vi "Auto Execute Commands.vi"(11 "Auto Commands":T1=[{"Drive Duration"=0.0, "Left Speed"=0.0, "Right Speed"=0.0, "Set Point"=1.0, "Set Point Duration"=2.0, "Command"=enum."Shooter", "Wait ms"=0.0}]) -> ()   [LabVIEW 2019]
uses:
  Controls/Auto Controls.ctl
  <vilib>/Rock Robotics/WPI/Solenoid/WPI_SolenoidValue.ctl
  <vilib>/Rock Robotics/WPI/Solenoid/WPI_SolenoidSetEnum.vi
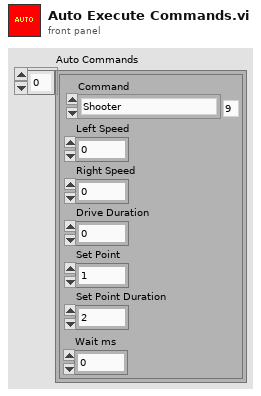
[diagram p1: front panel]
types:
  T1 = typedef "Auto Controls.ctl" = cluster{"Drive Duration":dbl, "Left Speed":dbl, "Right Speed":dbl, "Set Point":dbl, "Set Point Duration":dbl, "Command":enum16{"", "Drive Forwards", "Drive Backwards", "Stop", "Turn Left", "Turn Right", "Drop Intake", "Lift Intake", "Intake", "Shooter", "Transfer", "Wait"}, "Wait ms":dbl}[]
  T2 = typedef "WPI_SolenoidValue.ctl" = enum16{"Off", "On", "Forward", "Reverse"}
  T3 = enum16{"", "Drive Forwards", "Drive Backwards", "Stop", "Turn Left", "Turn Right", "Drop Intake", "Lift Intake", "Intake", "Shooter", "Transfer", "Wait"}
  T4 = typedef "WPI_SolenoidDevRef.ctl" = cluster{"DevStatus":errorcluster, "Pneumatics Control Module":u8, "Forward Solenoid Channel":T5, "Reverse Solenoid Channel":T5}
  T5 = typedef "WPI_SolenoidChannel.ctl" = enum8{"Solenoid 0", "Solenoid 1", "Solenoid 2", "Solenoid 3", "Solenoid 4", "Solenoid 5", "Solenoid 6", "Solenoid 7", "Invalid"}
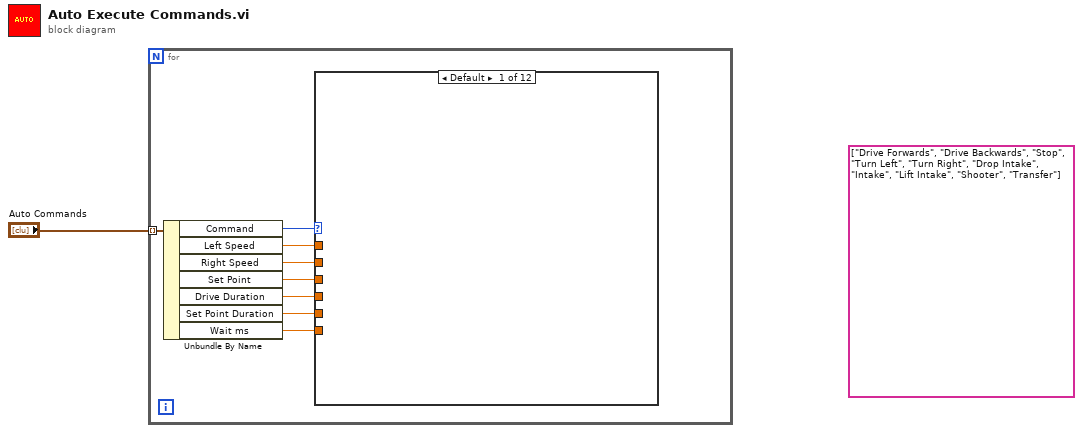
[diagram p0: block diagram]
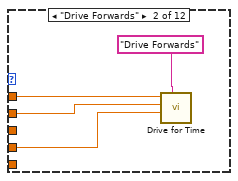
[diagram p2: hidden frame]
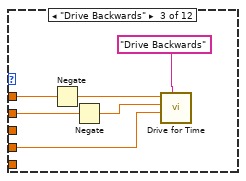
[diagram p3: hidden frame]
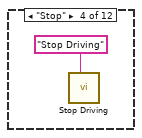
[diagram p4: hidden frame]
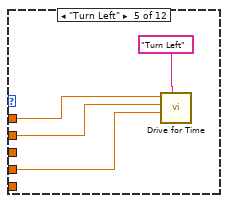
[diagram p5: hidden frame]
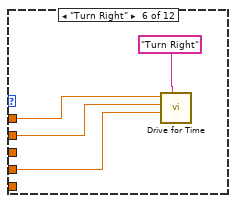
[diagram p6: hidden frame]
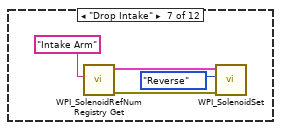
[diagram p7: hidden frame]
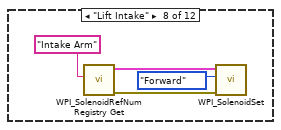
[diagram p8: hidden frame]
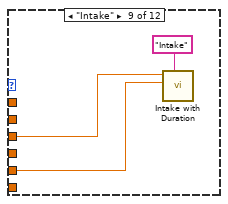
[diagram p9: hidden frame]
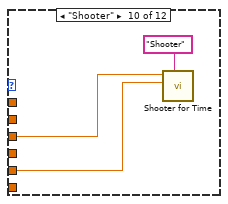
[diagram p10: hidden frame]
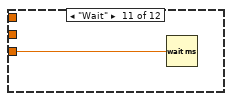
[diagram p11: hidden frame]
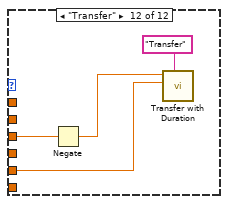
[diagram p12: hidden frame]
diagram:
  (unwired) string[] ["Drive Forwards", "Drive Backwards", "Stop", "Turn Left", "Turn Right", "Drop Intake", "Intake", "Lift Intake", "Shooter", "Transfer"]
  n1 = for {
    tunnel: "Auto Commands" -> [w9] mode=indexing
    n2 = Unbundle By Name(w9) -> ("Command"=w8:T3, "Left Speed"=w7:dbl, "Right Speed"=w6:dbl, "Set Point"=w4:dbl, "Drive Duration"=w5:dbl, "Set Point Duration"=w3:dbl, "Wait ms"=w2:dbl)
    n3 = case shown="Default" w8 {
      tunnel: w7 -> [_ w12 w18 _ w23 w27 _ _ _ _ _ _]
      tunnel: w6 -> [_ w11 w17 _ w22 w26 _ _ _ _ _ _]
      tunnel: w5 -> [_ w10 w16 _ w21 w25 _ _ _ _ _ _]
      tunnel: w4 -> [_ _ _ _ _ _ _ _ w38 w41 _ w46]
      tunnel: w3 -> [_ _ _ _ _ _ _ _ w37 w40 _ w44]
      tunnel: w2 -> [_ _ _ _ _ _ _ _ _ _ w43 _]
      frame Default {
      }
      frame "Drive Forwards" {
        n4 = call "Drive for Time.vi"("Description"="Drive Forwards", "Seconds"=w10, "Right Speed"=w11, "Left Speed"=w12) -> ()  [unwired: 7 in, 1 out]
      }
      frame "Drive Backwards" {
        n5 = Negate(x=w18) -> (-x=w15:dbl)
        n6 = Negate(x=w17) -> (-x=w14:dbl)
        n7 = call "Drive for Time.vi"("Description"="Drive Backwards", "Seconds"=w16, "Right Speed"=w14, "Left Speed"=w15) -> ()  [unwired: 7 in, 1 out]
      }
      frame "Stop" {
        n8 = call "Stop Driving.vi"("Description"="Stop Driving") -> ()  [unwired: 10 in, 1 out]
      }
      frame "Turn Left" {
        n9 = call "Drive for Time.vi"("Description"="Turn Left", "Seconds"=w21, "Right Speed"=w22, "Left Speed"=w23) -> ()  [unwired: 7 in, 1 out]
      }
      frame "Turn Right" {
        n10 = call "Drive for Time.vi"("Description"="Turn Right", "Seconds"=w25, "Right Speed"=w26, "Left Speed"=w27) -> ()  [unwired: 7 in, 1 out]
      }
      frame "Drop Intake" {
        n11 = call <vilib>:"WPI_SolenoidRefNum Registry Get.vi"("refnum name"="Intake Arm") -> ("error out"=w30:errorcluster, "SolenoidDevRef"=w31:T4)  [unwired: 9 in]
        n12 = call-poly <vilib>:"WPI_SolenoidSet.vi"("error in (no error)"=w30, "Value"=WPI_SolenoidValue."Reverse", "SolenoidDevRef"=w31) -> ()  [unwired: 7 in, 2 out]
      }
      frame "Lift Intake" {
        n13 = call <vilib>:"WPI_SolenoidRefNum Registry Get.vi"("refnum name"="Intake Arm") -> ("error out"=w34:errorcluster, "SolenoidDevRef"=w35:T4)  [unwired: 9 in]
        n14 = call-poly <vilib>:"WPI_SolenoidSet.vi"("error in (no error)"=w34, "Value"=WPI_SolenoidValue."Forward", "SolenoidDevRef"=w35) -> ()  [unwired: 7 in, 2 out]
      }
      frame "Intake" {
        n15 = call "Intake with Duration.vi"("Description"="Intake", "Duration (s)"=w37, "Setpoint"=w38) -> ()  [unwired: 8 in, 1 out]
      }
      frame "Shooter" {
        n16 = call "Shooter for Time.vi"("Description"="Shooter", "Duration (s)"=w40, "Setpoint"=w41) -> ()  [unwired: 8 in, 1 out]
      }
      frame "Wait" {
        n17 = Wait (ms)(milliseconds to wait=w43) -> ()  [unwired: 1 out]
      }
      frame "Transfer" {
        n18 = Negate(x=w46) -> (-x=w45:dbl)
        n19 = call "Transfer with Duration.vi"("Description"="Transfer", "Duration (s)"=w44, "Setpoint"=w45) -> ()  [unwired: 8 in, 1 out]
      }
    }
  }
